vi "禹山电导率校准.vi"() -> ()   [LabVIEW 2016, in "斯坦道多参数.lvlib"]
uses:
  <vilib>/Utility/miscctls.llb/LVPointTypeDef.ctl
  <vilib>/Analysis/NI_AALBase.lvlib
  <vilib>/Analysis/NI_AALPro.lvlib
  <vilib>/Utility/config.llb/NI_LVConfig.lvlib
panel:
  out "滤波设定":dbl
  out "盐度":dbl caption="盐度测量值" format="%#.2f"
  out "通讯状态":string
  out "第二点校准值":dbl
  out "第一点校准值":dbl
  out "最小值":sgl format="%.2g"
  out "最大值":sgl format="%.2g"
  in  "校准停止":bool
  in  "校准模式":u16(ring) items=["两点校准", "单点校准"]
  in  "标液2":dbl
  in  "标液1":dbl
  out "波形图表":sgl(graph) caption="历史曲线"
  out "温度测量值":dbl caption="温度" format="%#.2f"
  out "变异系数":dbl format="%.6g"
  out "standard deviation":dbl caption="标准差" format="%0.2f"
  out "mean":dbl caption="均值" format="%0.2f"
  out "提示":string
  in  "校准启动":bool
  out "测试值":dbl format="%#.2f"
  out "电极斜率":dbl format="%#.6f"
  out "电极零点":dbl format="%#.6f"
  # "电导率电极设定"
  # "℃"
  # "μS/cm"
  # "ppt"
  # "请选择校准模式:"
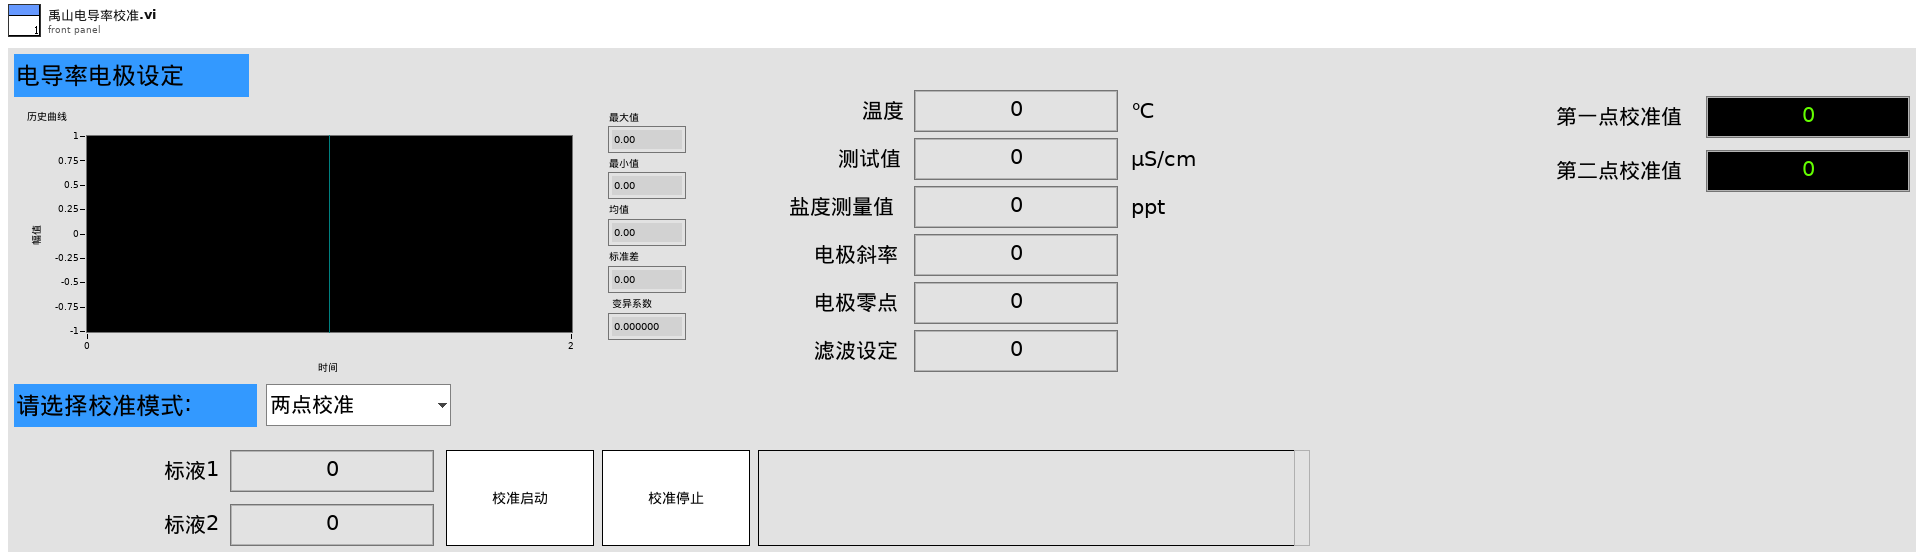
[diagram p1: front panel]
types:
  T1 = enum16{"pH", "DO", "Cond", "Turb", "ORP", "叶绿素a", "藻密度"}
  T2 = typedef "LVPointTypeDef.ctl" = cluster{"Horizontal":i16, "Vertical":i16}
  T3 = cluster{"pH":u32, "DO":u32, "Cond":u32, "Turb":u32, "叶绿素a":u32, "藻密度":u32, "ORP":u32, "COD":u32}
  T4 = typedef "NI_LVConfig.lvlib/Config Data RefNum.ctl" = refnum<k1>
  T5 = cluster{"温度测量值":sgl, "测量值":sgl, "温度偏移修正值":sgl, "信号值":sgl, "数据标识":string}
  T6 = enum8{"Enabled", "Disabled", "Disabled and Grayed Out"}
  T7 = cluster{"ph":bool, "DO":bool, "Cond":bool, "Turb":bool, "叶绿素a":bool, "藻密度":bool, "ORP":bool, "COD":bool}
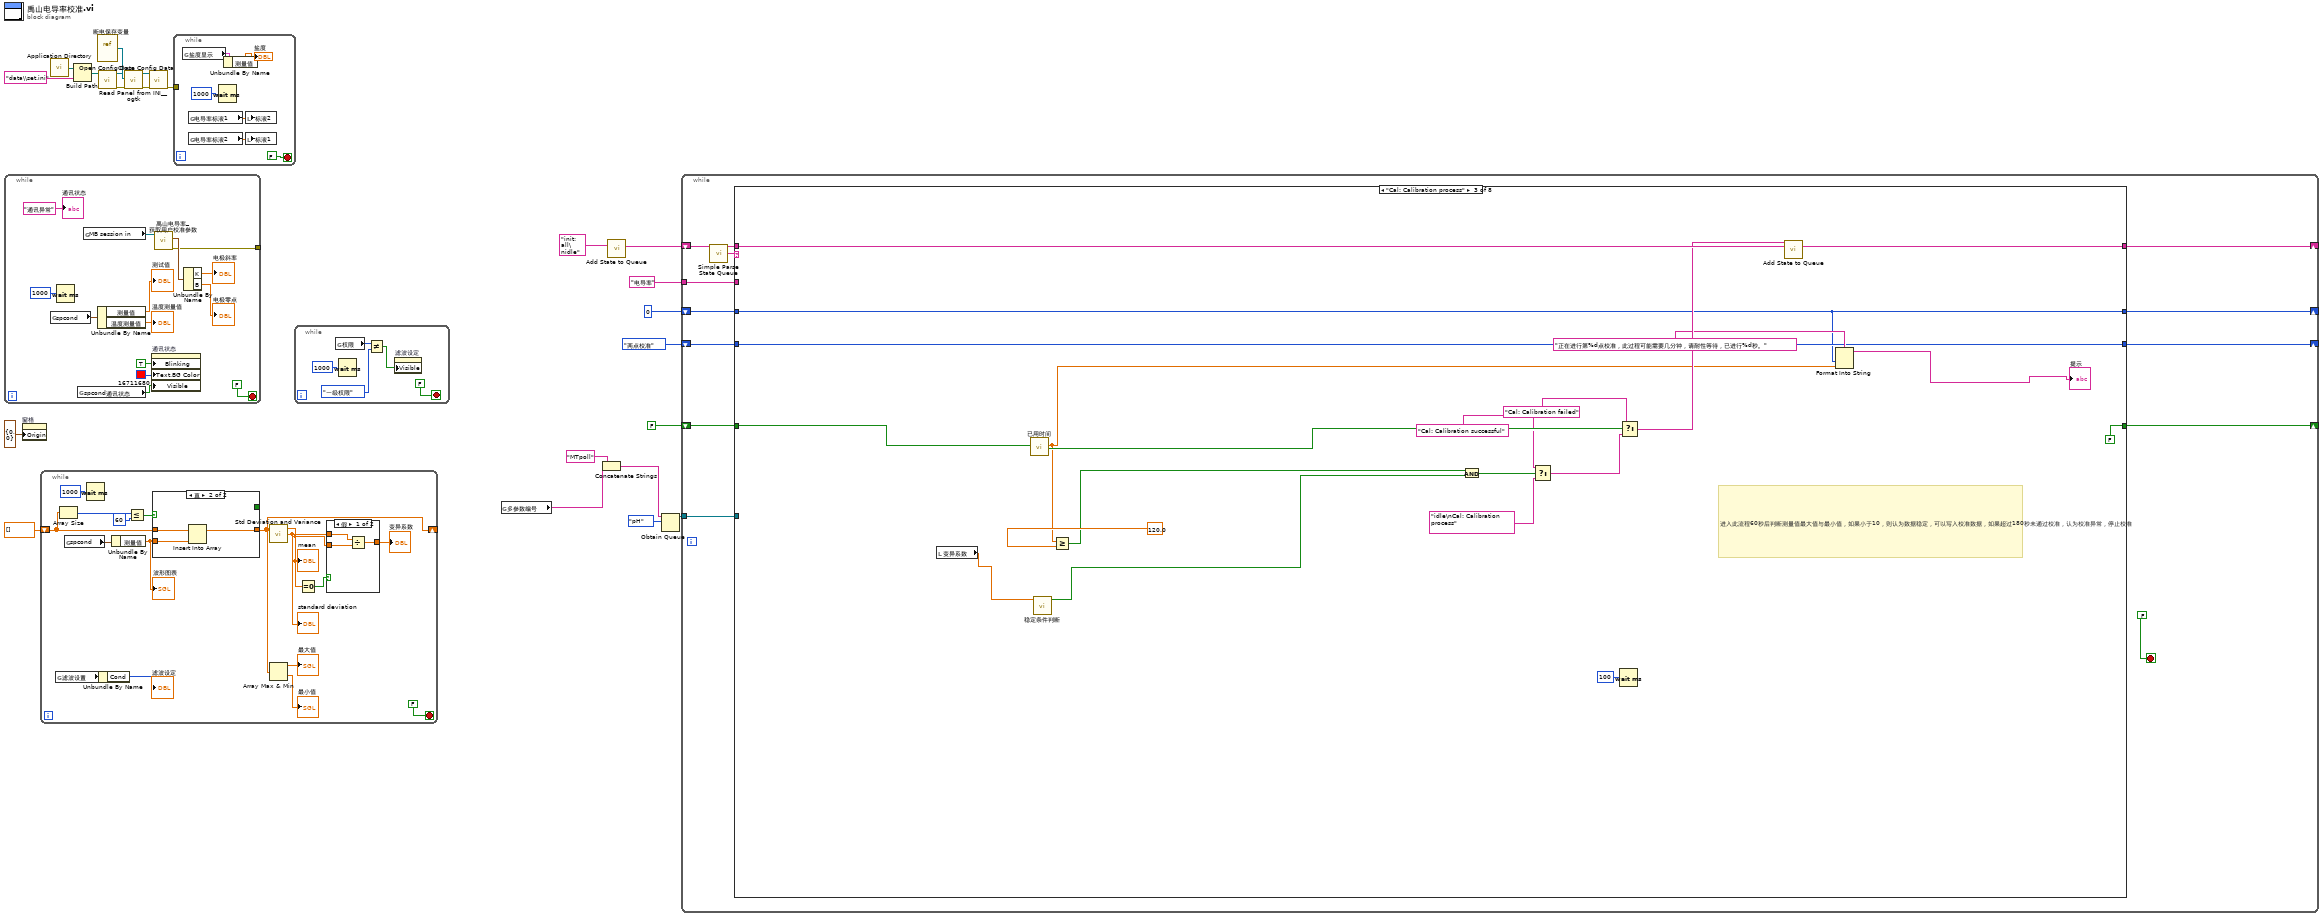
[diagram p0: block diagram]
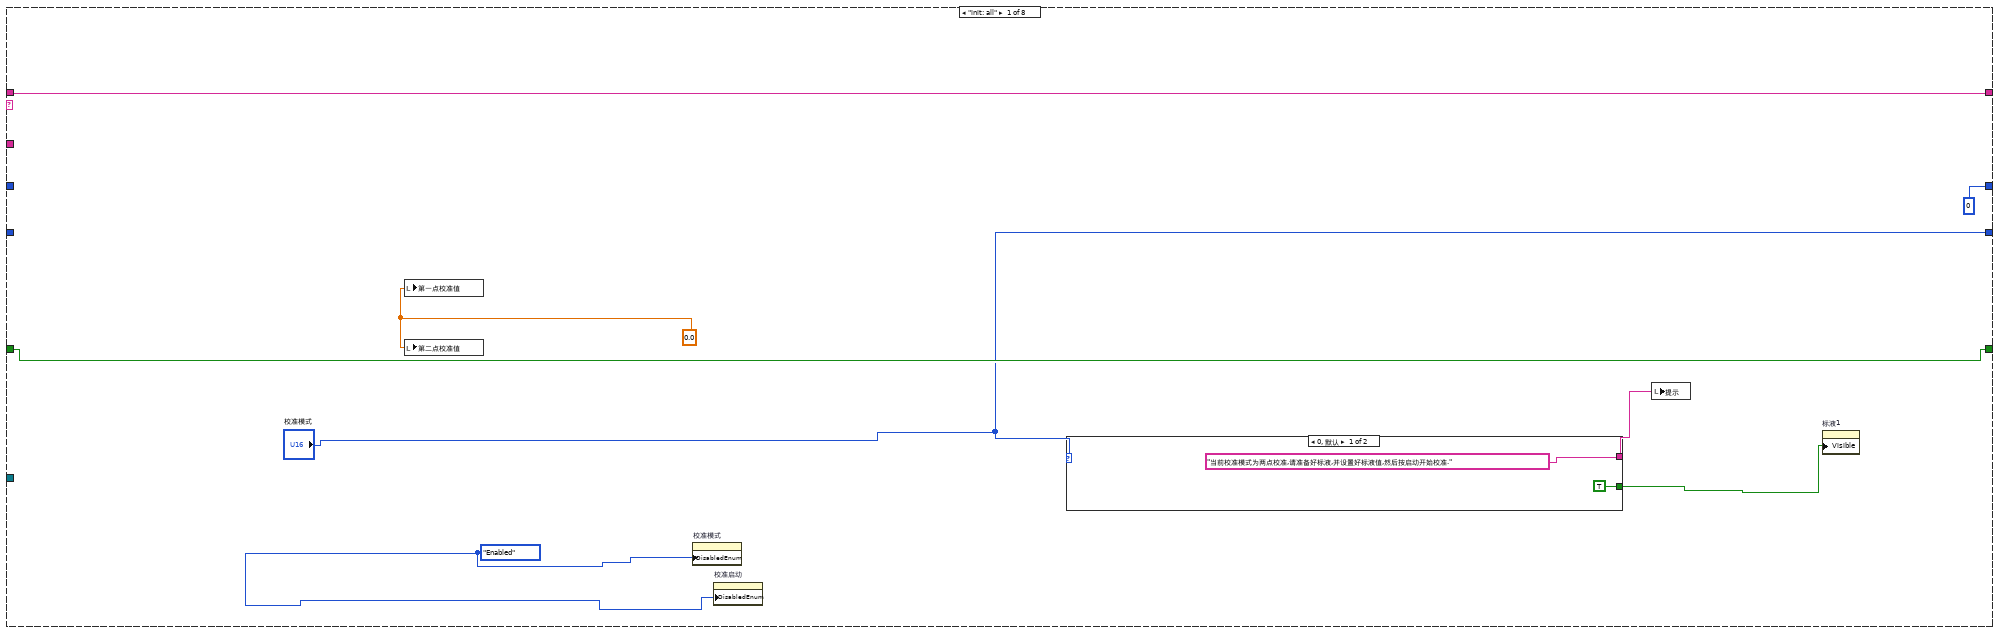
[diagram p2: hidden frame]
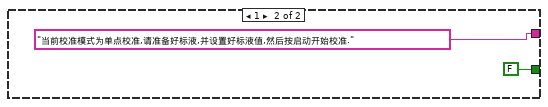
[diagram p3: hidden frame]
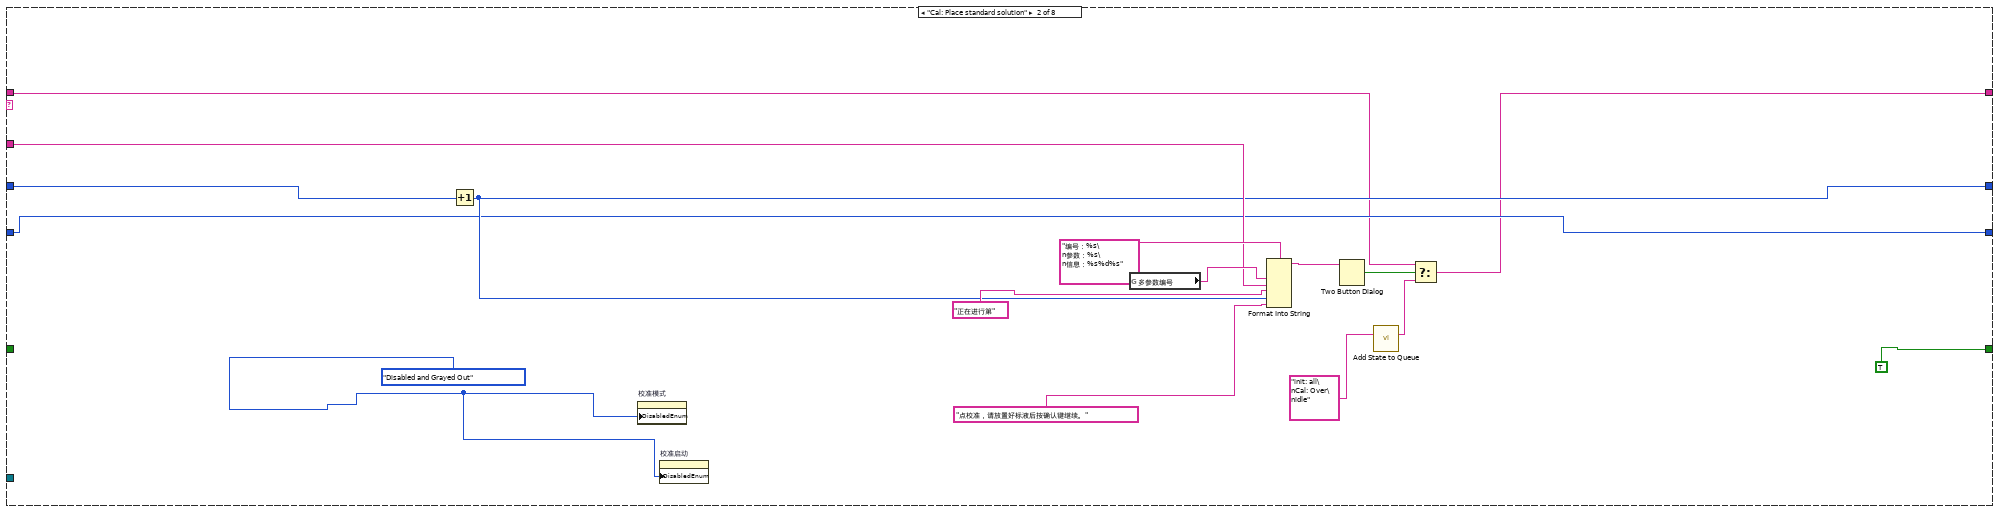
[diagram p4: hidden frame]
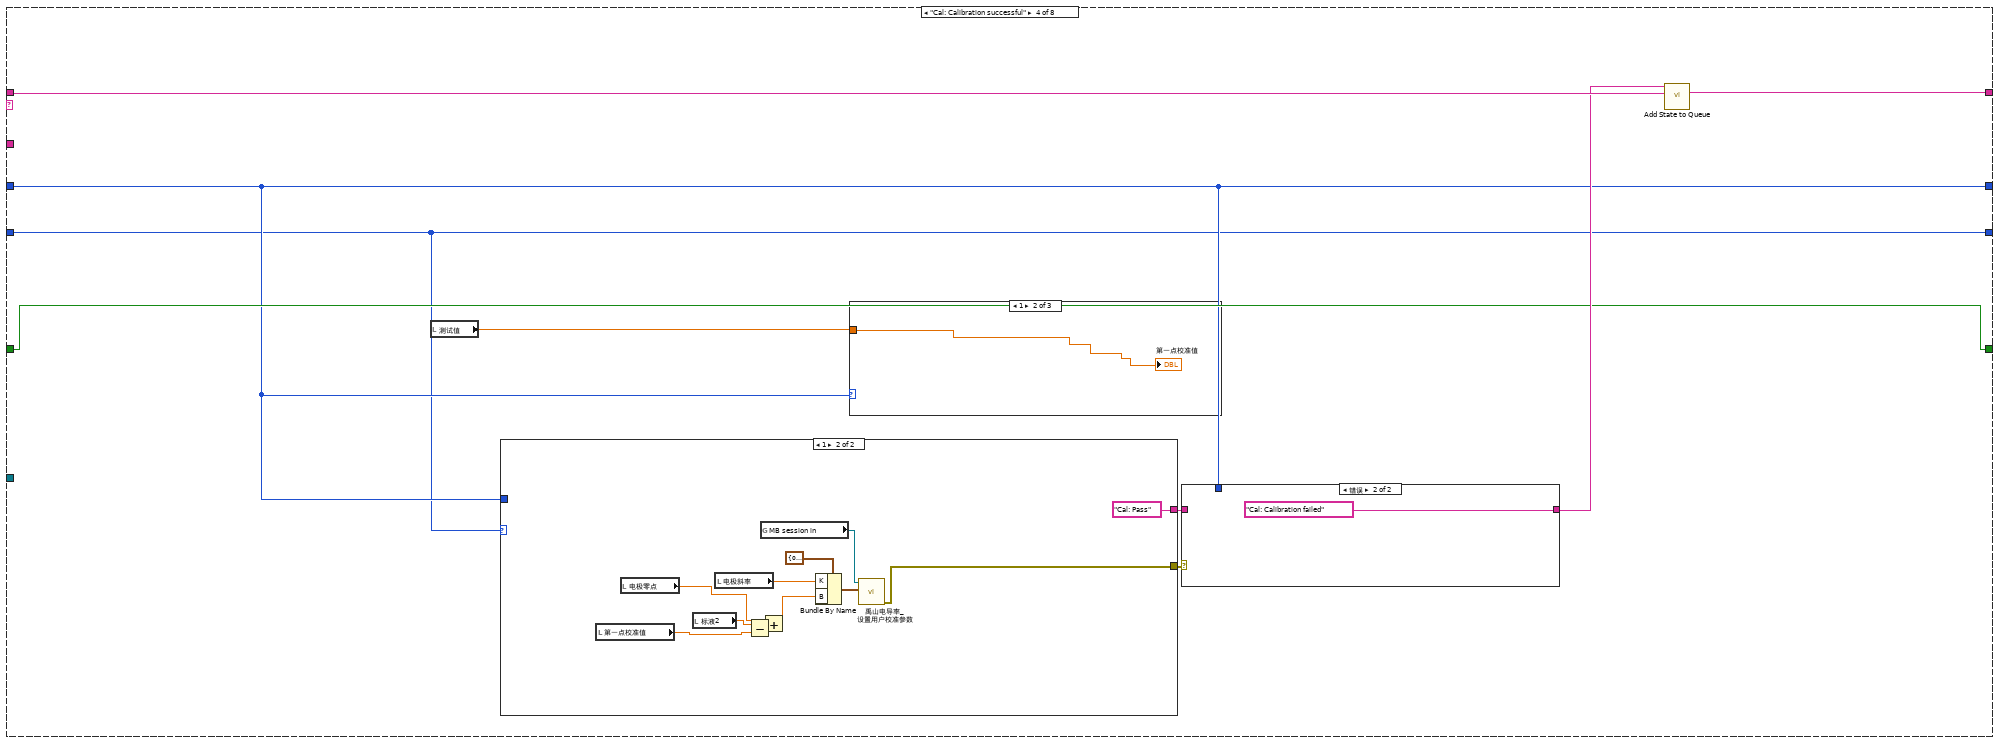
[diagram p5: hidden frame]
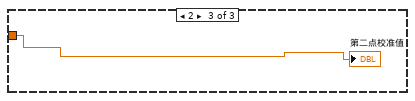
[diagram p7: hidden frame]
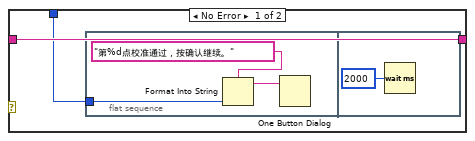
[diagram p8: hidden frame]
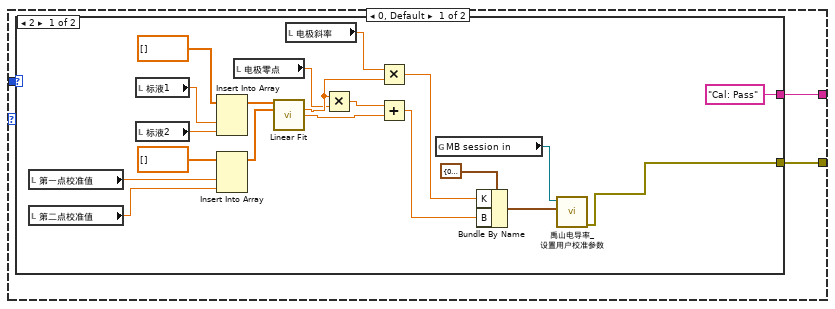
[diagram p9: hidden frame]
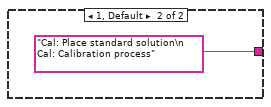
[diagram p10: hidden frame]
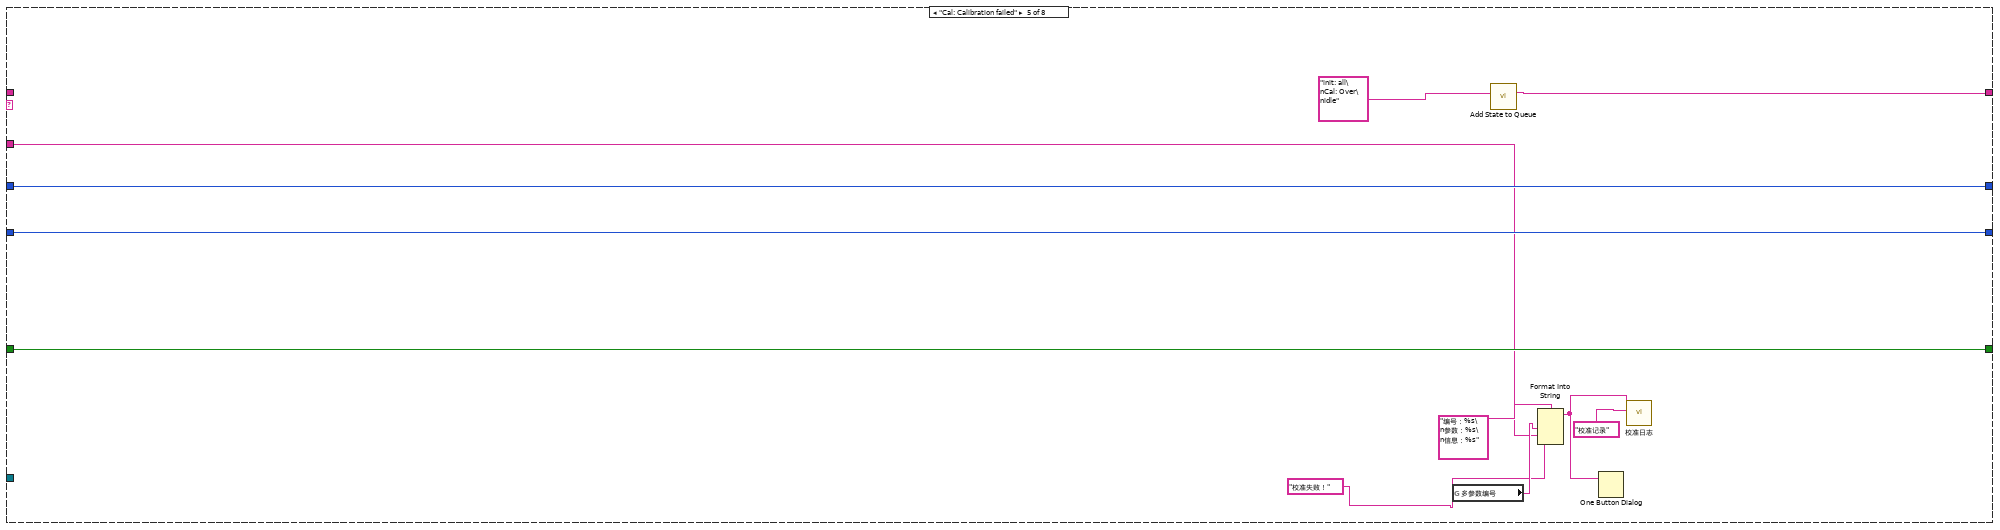
[diagram p11: hidden frame]
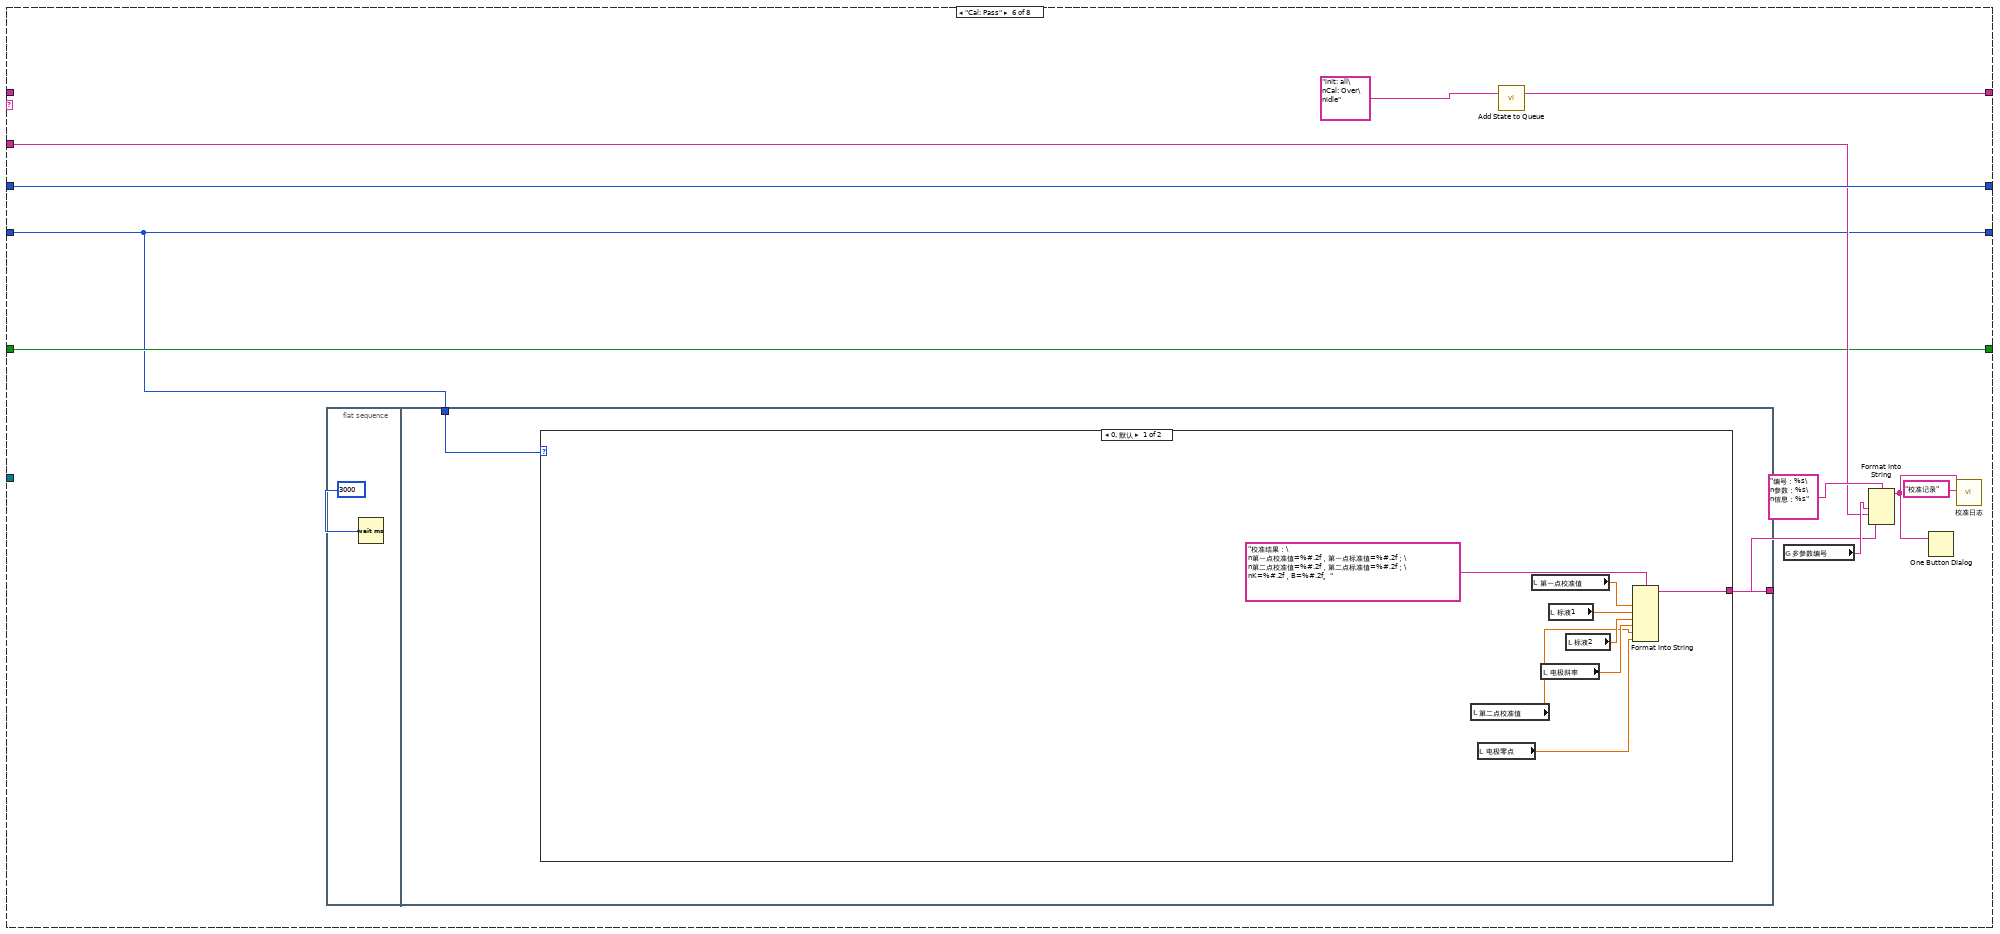
[diagram p12: hidden frame]
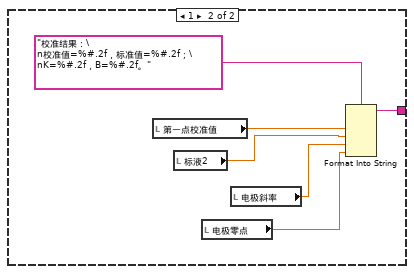
[diagram p13: hidden frame]
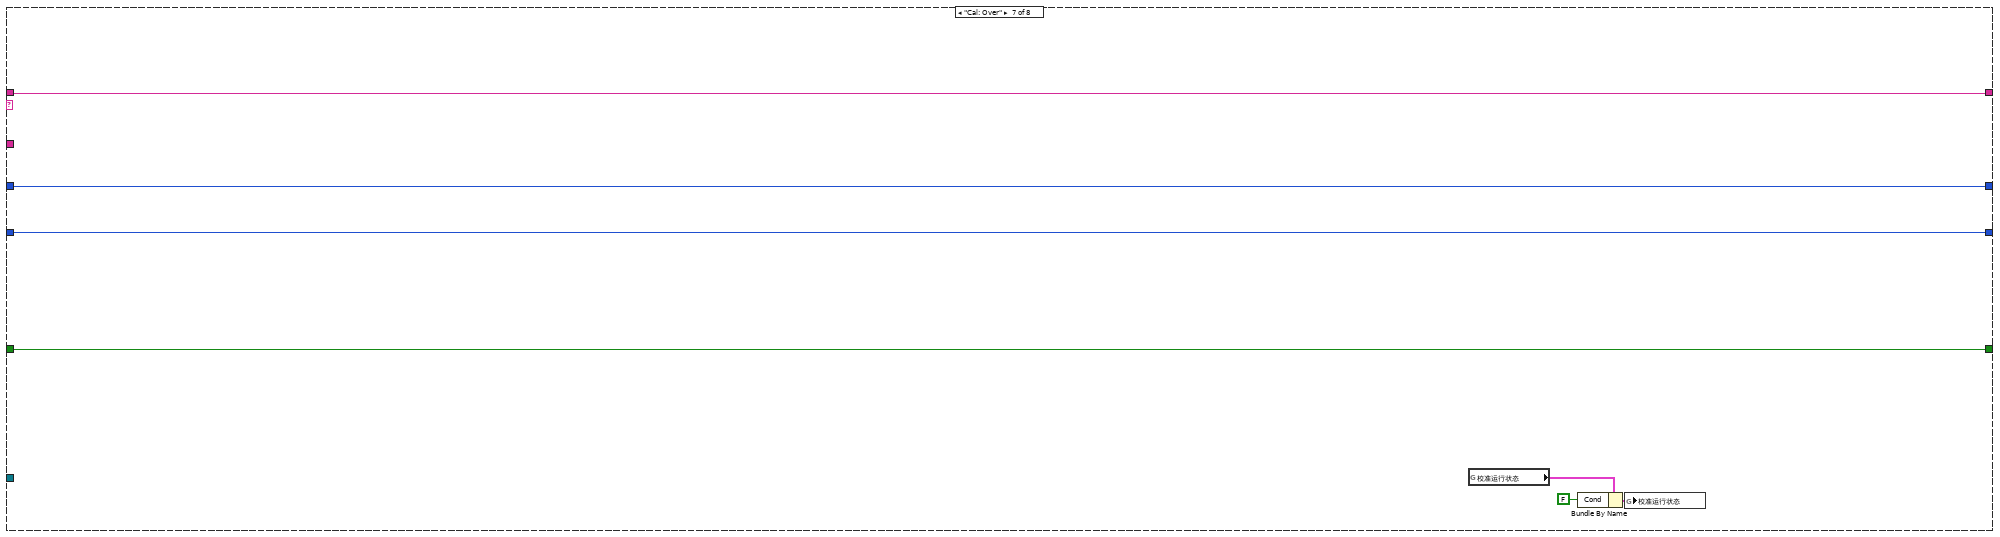
[diagram p14: hidden frame]
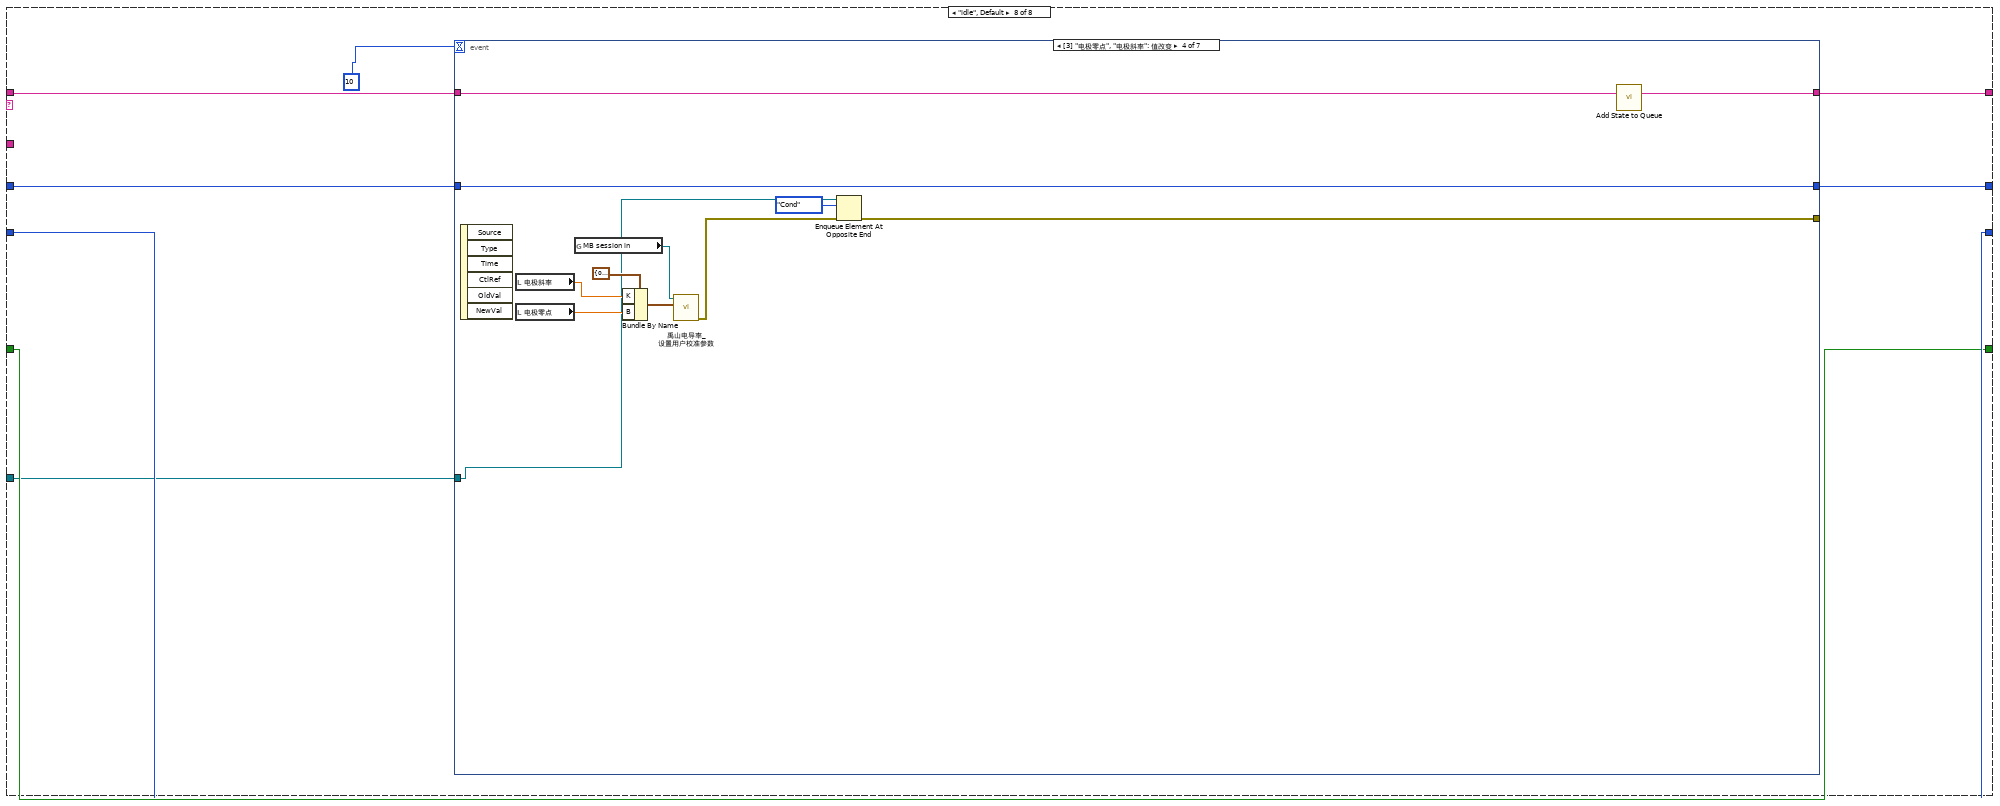
[diagram p15: hidden frame]
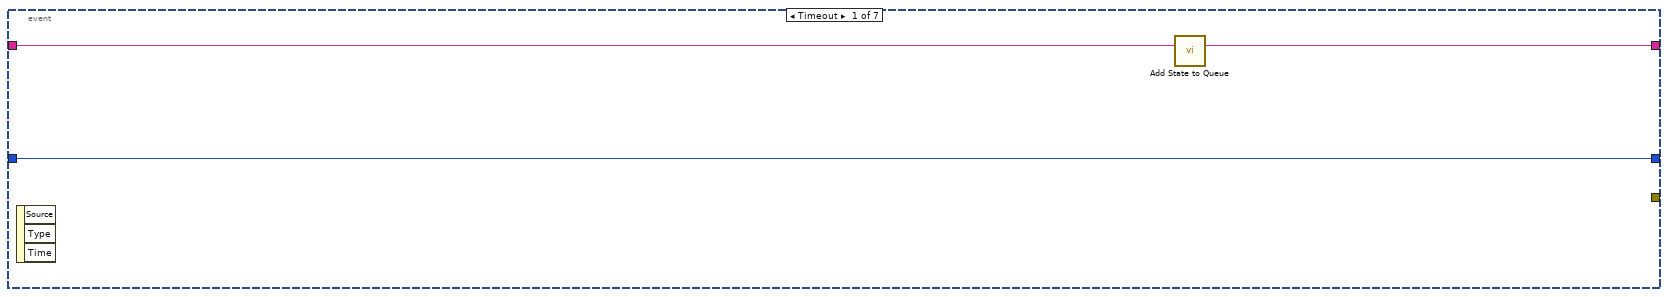
[diagram p16: hidden frame]
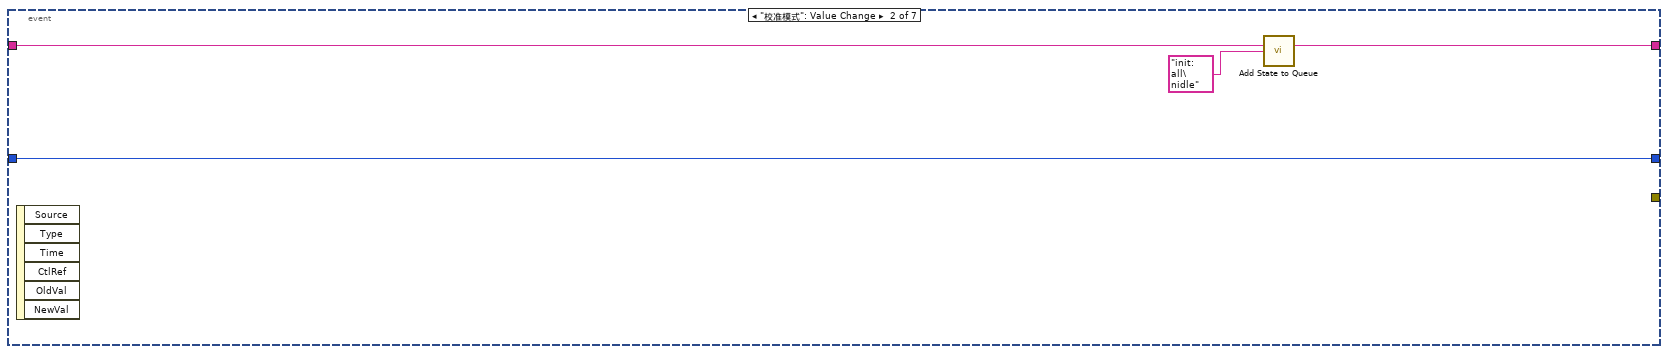
[diagram p17: hidden frame]
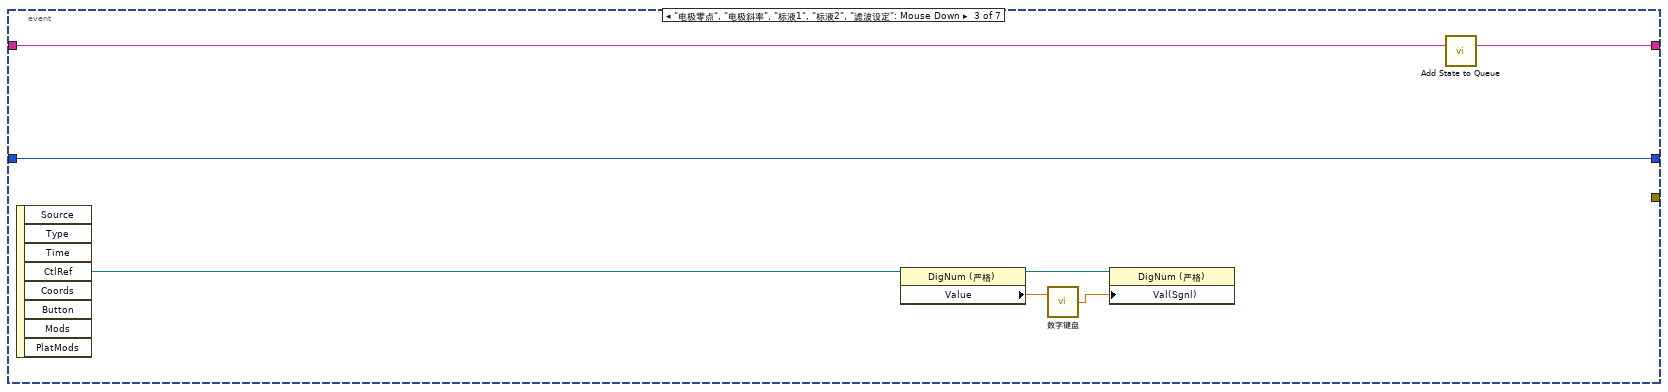
[diagram p18: hidden frame]
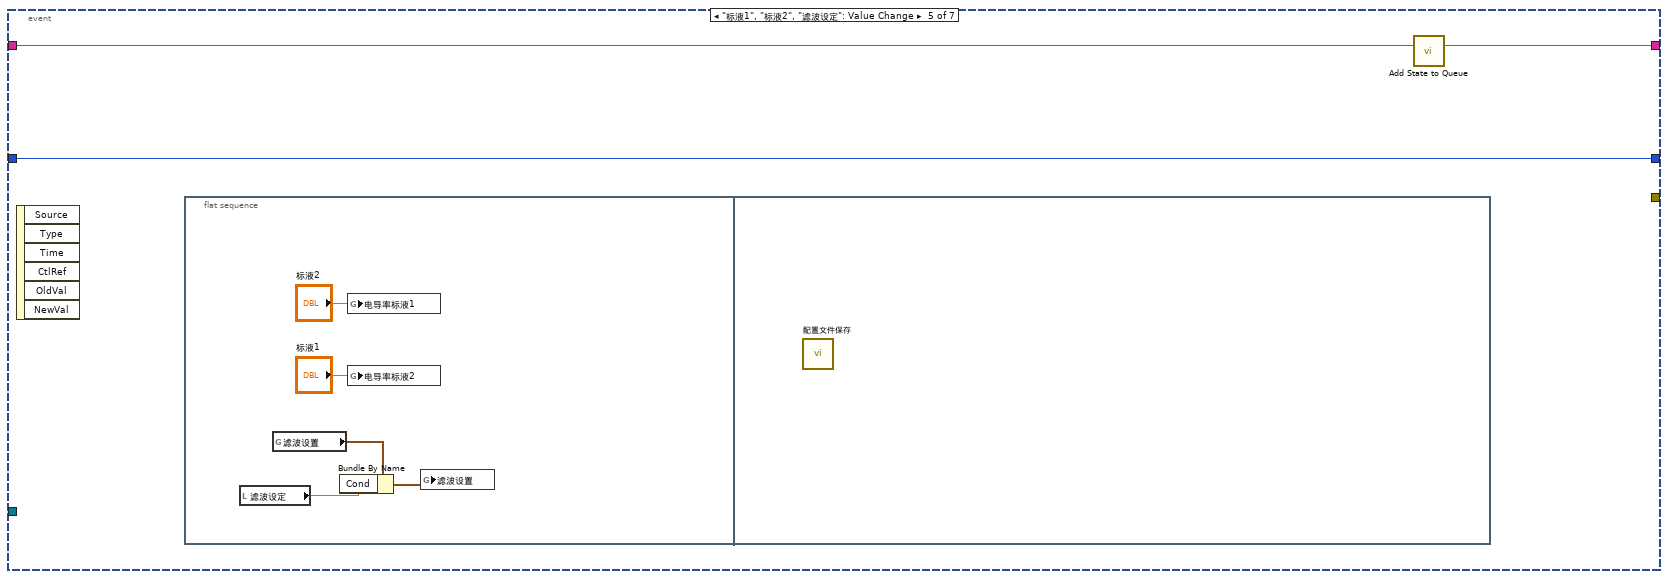
[diagram p19: hidden frame]
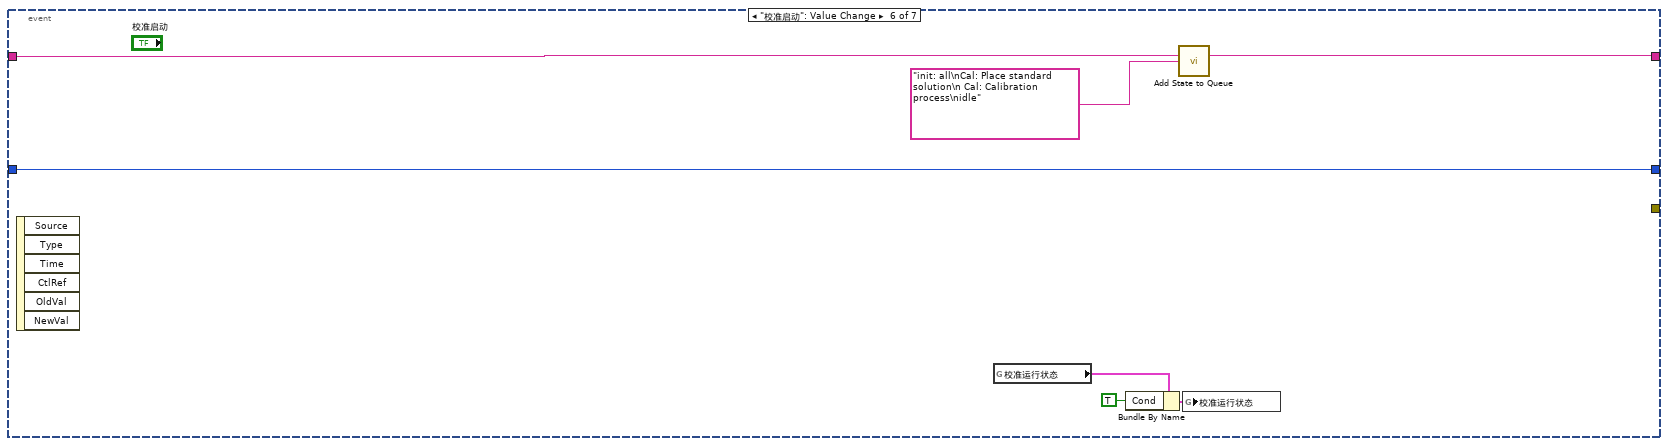
[diagram p20: hidden frame]
diagram:
  n1 = while {
    tunnel: [w31] -> _
    stop <- FALSE stop-if-true
    n2 = global read "禹山过程全局变量.vi" "spcond"() -> (w28:cluster{"温度测量值":sgl, "测量值":sgl, "错误标志":u16})
    n3 = Wait (ms)(milliseconds to wait=u32 1000 ("等待时间（毫秒）")) -> ()  [unwired: 1 out]
    n4 = global read "多参数全局变量.vi" "spcond通讯状态"() -> (w23:bool)
    n5 = global read "多参数全局变量.vi" "MB session in"() -> (w27:refnum<class "MB_Master.lvclass">)
    n6 = Unbundle By Name(w28) -> ("测量值"=→"测试值":sgl, "温度测量值"=→"温度测量值":sgl)
    n7 = property on="通讯状态" class="Str"("Blinking"=TRUE ("闪烁"), "Text.BG Color"=u32 16711680, "Visible"=w23) -> ()  [unwired: 2 in, 2 out]
    n8 = call "禹山电导率_获取用户校准参数.vi"("MB session in"=w27) -> ("error out"=w31:errorcluster, "输出值"=w34:cluster{"K":sgl, "B":sgl})  [unwired: 8 in, 1 out]
    n9 = Unbundle By Name(w34) -> ("K"=→"电极斜率":sgl, "B"=→"电极零点":sgl)
    "通讯状态" <- "通讯异常" ("当前串口")
  }
  n10 = property on="窗格" class="Pane"("Origin"=T2 {"Horizontal"=0, "Vertical"=0} ("原点")) -> ()  [unwired: 2 in, 2 out]
  n11 = while {
    shift-right: [w41] -> _
    shift-left: sgl[] [] -> [w49]
    stop <- FALSE stop-if-true
    n12 = global read "断电保存变量.vi" "滤波设置"() -> (w38:T3)
    n13 = Array Size(array=w49) -> (size(s)=w51:i32)
    n14 = global read "禹山过程全局变量.vi" "spcond"() -> (w43:cluster{"温度测量值":sgl, "测量值":sgl, "错误标志":u16})
    n15 = Wait (ms)(milliseconds to wait=u32 1000 ("等待时间（毫秒）")) -> ()  [unwired: 1 out]
    n16 = Unbundle By Name(w38) -> ("Cond"=→"滤波设定":u32)
    n17 = Unbundle By Name(w43) -> ("测量值"=w42:sgl)
    "波形图表" <- w42
    n18 = Less Or Equal?(x=w51, y=60) -> (x <= y?=w50:bool)
    n19 = case shown="真" w50 {
      tunnel: w49 -> [w62 w65]
      tunnel: w42 -> [w60 w64]
      tunnel: [w58 w63] -> w41
      tunnel: [TRUE _] -> _
      frame False {
        n20 = Replace Array Subset(array=w62, new element=w60) -> (w61:sgl[])  [unwired: 1 in]
        n21 = Rotate 1D Array(1:w61, 2:-1 ("n")) -> (0:w58:sgl[])
      }
      frame True {
        n22 = Insert Into Array(array=w65, new element=w64) -> (w63:sgl[])  [unwired: 1 in]
      }
    }
    n23 = call <vilib>:"Std Deviation and Variance.vi"("X"=w41) -> ("mean"=w44:dbl, "standard deviation"=w45:dbl)  [unwired: 1 in, 1 out]
    "standard deviation" <- w45
    "mean" <- w44
    n24 = Array Max & Min(array=w41) -> (max value=→"最大值":sgl, min value=→"最小值":sgl)  [unwired: 2 out]
    n25 = Equal To 0?(x=w44) -> (x = 0?=w48:bool)
    n26 = case shown="假" w48 {
      tunnel: w45 -> [w56 _]
      tunnel: [w55 _] -> w47
      tunnel: w44 -> [w54 _]
      frame False {
        n27 = Divide(x=w56, y=w54) -> (x/y=w55:dbl)
      }
      frame True {
      }
    }
    "变异系数" <- w47
  }
  n28 = call <vilib>:"Application Directory.vi"() -> ("Application Directory"=w17:path)
  n29 = Build Path(base path=w17, name or relative path="data\\set.ini" ("名称或相对路径")) -> (appended path=w18:path)
  n30 = vi-ref "断电保存变量.vi"() -> (w20:refnum<vi>)
  n31 = call <vilib>:"Open Config Data.vi"("configuration file path"=w18) -> ("error out"=w14:errorcluster, "refnum"=w13:T4)  [unwired: 8 in, 1 out]
  n32 = call <userlib>:"Read Panel from INI__ogtk.vi"("error in (no error)"=w14, "VI ref"=w20, "refnum"=w13) -> ("error out"=w16:errorcluster, "refnum out"=w15:T4)  [unwired: 7 in]
  n33 = call <vilib>:"Close Config Data.vi"("error in (no error)"=w16, "refnum"=w15) -> ("error out"=w12:errorcluster)  [unwired: 8 in, 1 out]
  n34 = while {
    tunnel: w12 -> [_]
    stop <- FALSE stop-if-true
    n35 = global read "多参数全局变量.vi" "盐度显示"() -> (w67:T5)
    n36 = global read "断电保存变量.vi" "电导率标液1"() -> (w68:dbl)
    n37 = global read "断电保存变量.vi" "电导率标液2"() -> (w69:dbl)
    n38 = Wait (ms)(milliseconds to wait=u32 1000 ("等待时间（毫秒）")) -> ()  [unwired: 1 out]
    n39 = Unbundle By Name(w67) -> ("测量值"=→"盐度":sgl)
    n40 = local write "标液2"(w68) -> ()
    n41 = local write "标液1"(w69) -> ()
  }
  n42 = while {
    stop <- FALSE stop-if-true
    n43 = global read "多参数全局变量.vi" "权限"() -> (w75:enum16{"一级权限", "二级权限", "三级权限"})
    n44 = Wait (ms)(milliseconds to wait=u32 1000 ("等待时间（毫秒）")) -> ()  [unwired: 1 out]
    n45 = Not Equal?(x=w75, y=enum16{"一级权限", "二级权限", "三级权限"}."一级权限") -> (x != y?=w72:bool)
    n46 = property on="滤波设定" class="DigNum (严格)"("Visible"=w72) -> ()  [unwired: 2 in, 2 out]
  }
  n47 = global read "多参数全局变量.vi" "多参数编号"() -> (w2:string)
  n48 = Concatenate Strings("MTpoll" ("名称（未命名）"), w2) -> (w4:string)
  n49 = call "Add State to Queue.vi"("State(s) In (\"\")"="init: all\nidle" ("State(s) In (\"\")")) -> ("States Out"=w10:string)  [unwired: 14 in]
  n50 = Obtain Queue(name (unnamed)=w4, element data type=T1."pH" ("枚举")) -> (queue out=w1:refnum<queue>)  [unwired: 3 in, 2 out]
  n51 = while {
    shift-right: [w85] -> _
    shift-left: w10 -> [w89]
    shift-right: [w82] -> _
    shift-left: 0 -> [w84]
    tunnel: "电导率" ("State(s) In (\"\")") -> [w83]
    shift-right: [w80] -> _
    shift-left: enum16{"两点校准", "单点校准"}."两点校准" ("校准模式") -> [w81]
    shift-right: [w78] -> _
    shift-left: FALSE -> [w79]
    tunnel: w1 -> [w77]
    stop <- FALSE stop-if-true
    n52 = call "Simple Parse State Queue.vi"("State Queue"=w89) -> ("Remain States"=w86:string, "Next State"=w87:string)  [unwired: 13 in]
    n53 = case shown="\"Cal: Calibration process\"" w87 {
      tunnel: w86 -> [w97 w105 w137 w145 _ _ w234 w245]
      tunnel: [w97 w104 w136 w144 w199 w204 w234 w244] -> w85
      tunnel: w84 -> [_ w113 w122 w140 w202 w213 w233 w242]
      tunnel: w83 -> [_ w114 _ _ w193 w209 _ _]
      tunnel: [0 w111 w122 w140 w202 w213 w233 w243] -> w82
      tunnel: w81 -> [_ w110 w123 w139 w201 w205 w232 w241]
      tunnel: ["校准模式" w110 w123 w139 w201 w205 w232 w241] -> w80
      tunnel: w79 -> [w94 _ w125 w141 w200 w208 w231 w239]
      tunnel: [w94 TRUE FALSE w141 w200 w208 w231 w239] -> w78
      tunnel: w77 -> [_ _ _ _ _ _ _ w238]
      frame "init: all" {
        w91 = T6."Enabled" ("禁用")
        w93 = 0.0 ("第一点校准值")
        n54 = local write "第一点校准值"(w93) -> ()
        n55 = local write "第二点校准值"(w93) -> ()
        n56 = property on="校准模式" class="Ring (严格)"("DisabledEnum"=w91) -> ()  [unwired: 2 in, 2 out]
        n57 = property on="校准启动" class="Bool"("DisabledEnum"=w91) -> ()  [unwired: 2 in, 2 out]
        n58 = case shown="0, 默认" "校准模式" {
          tunnel: ["当前校准模式为两点校准,请准备好标液,并设置好标液值,然后按启动开始校准." ("提示") "当前校准模式为单点校准,请准备好标液,并设置好标液值,然后按启动开始校准." ("提示")] -> w96
          tunnel: [TRUE ("可见") FALSE ("可见")] -> w90
          frame 0, Default {
          }
          frame 1 {
          }
        }
        n59 = local write "提示"(w96) -> ()
        n60 = property on="标液1" class="DigNum (严格)"("Visible"=w90) -> ()  [unwired: 2 in, 2 out]
      }
      frame "Cal: Place standard solution" {
        w103 = T6."Disabled and Grayed Out" ("禁用")
        n61 = Increment(x=w113) -> (x+1=w111:i32)
        n62 = property on="校准模式" class="Ring (严格)"("DisabledEnum"=w103) -> ()  [unwired: 2 in, 2 out]
        n63 = property on="校准启动" class="Bool"("DisabledEnum"=w103) -> ()  [unwired: 2 in, 2 out]
        n64 = global read "多参数全局变量.vi" "多参数编号"() -> (w116:string)
        n65 = Format Into String(format string="编号：%s\n参数：%s\n信息：%s%d%s" ("格式字符串"), w116, w114, "正在进行第" ("消息"), w111, "点校准，请放置好标液后按确认键继续。" ("消息")) -> (resulting string=w108:string)  [unwired: 2 in, 1 out]
        n66 = Two Button Dialog(message=w108) -> (T button?=w107:bool)  [unwired: 2 in]
        n67 = call "Add State to Queue.vi"("State(s) In (\"\")"="init: all\nCal: Over\nidle" ("State(s) In (\"\")")) -> ("States Out"=w106:string)  [unwired: 14 in]
        n68 = Select(t=w105, s=w107, f=w106) -> (s? t:f=w104:string)
      }
      frame "Cal: Calibration process" {
        # "进入此流程60秒后判断测量值最大值与最小值，如果小于10，则认为数据稳定，可以写入校准数据，如果超过180秒未通过校准，认为校准异常，停止校准"
        n69 = local read "变异系数"() -> (w119:dbl)
        n70 = call "已用时间"("Reset"=w125) -> ("Elapsed Time (s)"=w121:dbl, "Time has Elapsed"=w138:bool)  [unwired: 11 in, 6 out]
        n71 = call "稳定条件判断.vi"("变异系数"=w119) -> ("布尔"=w118:bool)  [unwired: 10 in]
        n72 = Greater Or Equal?(x=w121, y=120.0) -> (x >= y?=w133:bool)
        n73 = And(x=w133, y=w118) -> (x .and. y?=w130:bool)
        n74 = Select(t="Cal: Calibration successful" ("State(s) In (\"\")"), s=w130, f="idle\nCal: Calibration process" ("State(s) In (\"\")")) -> (s? t:f=w129:string)
        n75 = Wait (ms)(milliseconds to wait=u32 100 ("等待时间（毫秒）")) -> ()  [unwired: 1 out]
        n76 = Select(t="Cal: Calibration failed" ("State(s) In (\"\")"), s=w138, f=w129) -> (s? t:f=w128:string)
        n77 = call "Add State to Queue.vi"("State(s) In Front (\"\")"=w128, "State(s) In (\"\")"=w137) -> ("States Out"=w136:string)  [unwired: 13 in]
        n78 = Format Into String(format string="正在进行第%d点校准，此过程可能需要几分钟，请耐性等待，已进行%d秒。" ("格式字符串"), w122, w121) -> (resulting string=→"提示":string)  [unwired: 2 in, 1 out]
      }
      frame "Cal: Calibration successful" {
        n79 = local read "测试值"() -> (w142:dbl)
        n80 = case shown="1" w139 {
          tunnel: [w159 w181] -> w147
          tunnel: [w158 "Cal: Pass" ("State(s) In (\"\")")] -> w146
          tunnel: w140 -> [w157 _]
          frame 0, Default {
            n81 = case shown="2" w157 {
              tunnel: [w160 _] -> w159
              tunnel: ["Cal: Pass" ("State(s) In (\"\")") "Cal: Place standard solution\n Cal: Calibration process" ("State(s) In (\"\")")] -> w158
              frame 2 {
                n82 = local read "第一点校准值"() -> (w177:dbl)
                n83 = local read "第二点校准值"() -> (w176:dbl)
                n84 = local read "标液1"() -> (w174:dbl)
                n85 = local read "标液2"() -> (w173:dbl)
                n86 = Insert Into Array(array=dbl[] [] ("Weight"), new element #1=w174, new element #2=w173) -> (w172:dbl[])  [unwired: 1 in]
                n87 = Insert Into Array(array=dbl[] [] ("Weight"), new element #1=w177, new element #2=w176) -> (w171:dbl[])  [unwired: 1 in]
                n88 = local read "电极零点"() -> (w164:dbl)
                n89 = call <vilib>:"Linear Fit.vi"("Y"=w172, "X"=w171) -> ("slope"=w165:dbl, "intercept"=w162:dbl)  [unwired: 9 in, 3 out]
                n90 = local read "电极斜率"() -> (w167:dbl)
                n91 = Multiply(x=w165, y=w164) -> (x*y=w163:dbl)
                n92 = Multiply(x=w167, y=w165) -> (x*y=w166:dbl)
                n93 = Add(x=w163, y=w162) -> (x+y=w161:dbl)
                n94 = global read "多参数全局变量.vi" "MB session in"() -> (w170:refnum<class "MB_Master.lvclass">)
                n95 = Bundle By Name(cluster=cluster{"K":sgl, "B":sgl} {"K"=0.0, "B"=0.0} ("用户校准参数"), "K"=w166, "B"=w161) -> (w169:cluster{"K":sgl, "B":sgl})
                n96 = call "禹山电导率_设置用户校准参数.vi"("用户校准参数"=w169, "MB session in"=w170) -> ("error out"=w160:errorcluster)  [unwired: 8 in, 1 out]
              }
              frame 1, Default {
              }
            }
          }
          frame 1 {
            n97 = local read "第一点校准值"() -> (w186:dbl)
            n98 = local read "电极零点"() -> (w182:dbl)
            n99 = local read "标液2"() -> (w185:dbl)
            n100 = local read "电极斜率"() -> (w187:dbl)
            n101 = Subtract(x=w185, y=w186) -> (x-y=w184:dbl)
            n102 = global read "多参数全局变量.vi" "MB session in"() -> (w190:refnum<class "MB_Master.lvclass">)
            n103 = Add(x=w182, y=w184) -> (x+y=w183:dbl)
            n104 = Bundle By Name(cluster=cluster{"K":sgl, "B":sgl} {"K"=0.0, "B"=0.0} ("用户校准参数"), "K"=w187, "B"=w183) -> (w189:cluster{"K":sgl, "B":sgl})
            n105 = call "禹山电导率_设置用户校准参数.vi"("用户校准参数"=w189, "MB session in"=w190) -> ("error out"=w181:errorcluster)  [unwired: 8 in, 1 out]
          }
        }
        n106 = case shown="1" w140 {
          tunnel: w142 -> [_ w148 w149]
          frame 0, Default {
          }
          frame 1 {
            "第一点校准值" <- w148
          }
          frame 2 {
            "第二点校准值" <- w149
          }
        }
        n107 = case shown="错误" w147 {
          tunnel: w146 -> [w151 _]
          tunnel: [w151 "Cal: Calibration failed" ("State(s) In (\"\")")] -> w143
          tunnel: w140 -> [w150 _]
          frame No Error {
            n108 = flat-sequence {
              tunnel: w150 -> [w152]
              frame #0 {
                n109 = Format Into String(format string="第%d点校准通过，按确认继续。" ("格式字符串"), w152) -> (resulting string=w154:string)  [unwired: 2 in, 1 out]
                n110 = One Button Dialog(message=w154) -> ()  [unwired: 1 in, 1 out]
              }
              frame #1 {
                n111 = Wait (ms)(milliseconds to wait=u32 2000 ("等待时间（毫秒）")) -> ()  [unwired: 1 out]
              }
            }
          }
          frame Error {
          }
        }
        n112 = call "Add State to Queue.vi"("State(s) In Front (\"\")"=w143, "State(s) In (\"\")"=w145) -> ("States Out"=w144:string)  [unwired: 13 in]
      }
      frame "Cal: Calibration failed" {
        n113 = global read "多参数全局变量.vi" "多参数编号"() -> (w196:string)
        n114 = call "Add State to Queue.vi"("State(s) In (\"\")"="init: all\nCal: Over\nidle" ("State(s) In (\"\")")) -> ("States Out"=w199:string)  [unwired: 14 in]
        n115 = Format Into String(format string="编号：%s\n参数：%s\n信息：%s" ("格式字符串"), w196, w193, "校准失败！" ("消息")) -> (resulting string=w195:string)  [unwired: 2 in, 1 out]
        n116 = One Button Dialog(message=w195) -> ()  [unwired: 1 in, 1 out]
        n117 = call "校准日志.vi"("table"="校准记录", "日志信息"=w195) -> ()  [unwired: 9 in, 1 out]
      }
      frame "Cal: Pass" {
        n118 = flat-sequence {
          tunnel: [w216] -> w206
          tunnel: w205 -> [w215]
          frame #0 {
            n119 = Wait (ms)(milliseconds to wait=u32 3000 ("等待时间（毫秒）")) -> ()  [unwired: 1 out]
          }
          frame #1 {
            n120 = case shown="0, 默认" w215 {
              tunnel: [w224 w230] -> w216
              frame 0, Default {
                n121 = local read "第二点校准值"() -> (w218:dbl)
                n122 = local read "电极零点"() -> (w217:dbl)
                n123 = local read "第一点校准值"() -> (w222:dbl)
                n124 = local read "电极斜率"() -> (w219:dbl)
                n125 = local read "标液1"() -> (w223:dbl)
                n126 = local read "标液2"() -> (w220:dbl)
                n127 = Format Into String(format string="校准结果：\n第一点校准值=%#.2f，第一点标准值=%#.2f；\n第二点校准值=%#.2f，第二点标准值=%#.2f；\nK=%#.2f，B=%#.2f。" ("提示"), w222, w223, w220, w219, w218, w217) -> (resulting string=w224:string)  [unwired: 2 in, 1 out]
              }
              frame 1 {
                n128 = local read "第一点校准值"() -> (w229:dbl)
                n129 = local read "标液2"() -> (w227:dbl)
                n130 = local read "电极零点"() -> (w225:dbl)
                n131 = local read "电极斜率"() -> (w226:dbl)
                n132 = Format Into String(format string="校准结果：\n校准值=%#.2f，标准值=%#.2f；\nK=%#.2f，B=%#.2f。" ("提示"), w229, w227, w226, w225) -> (resulting string=w230:string)  [unwired: 2 in, 1 out]
              }
            }
          }
        }
        n133 = call "Add State to Queue.vi"("State(s) In (\"\")"="init: all\nCal: Over\nidle" ("State(s) In (\"\")")) -> ("States Out"=w204:string)  [unwired: 14 in]
        n134 = global read "多参数全局变量.vi" "多参数编号"() -> (w210:string)
        n135 = Format Into String(format string="编号：%s\n参数：%s\n信息：%s" ("格式字符串"), w210, w209, w206) -> (resulting string=w207:string)  [unwired: 2 in, 1 out]
        n136 = One Button Dialog(message=w207) -> ()  [unwired: 1 in, 1 out]
        n137 = call "校准日志.vi"("table"="校准记录", "日志信息"=w207) -> ()  [unwired: 9 in, 1 out]
      }
      frame "Cal: Over" {
        n138 = global read "多参数全局变量.vi" "校准运行状态"() -> (w236:T7)
        n139 = Bundle By Name(cluster=w236, "Cond"=FALSE) -> (w237:T7)
        n140 = global write "多参数全局变量.vi" "校准运行状态"(w237) -> ()
      }
      frame "idle", Default {
        n141 = event shown="[3] \"电极零点\", \"电极斜率\": 值改变" {
          selector: _ -> [_ _ _ _ _ _ _]
          dyn-events: _ -> [_ _ _ _ _ _ _]
          timeout: 10 -> [_ _ _ _ _ _ _]
          tunnel: [_ _ _ w262 _ _ _] -> _
          tunnel: w245 -> [w248 w252 w257 w263 w272 w286 _]
          tunnel: [w247 w251 w258 w270 w273 w285 w288] -> w244
          tunnel: [w246 w249 w259 w271 w274 w283 w289] -> w243
          tunnel: w242 -> [w246 w249 w259 w271 w274 w283 w289]
          tunnel: w238 -> [_ _ _ w261 _ _ _]
          event Timeout {
            n142 = event-data() -> ()  [unwired: 1 in, 3 out]
            n143 = call "Add State to Queue.vi"("State(s) In (\"\")"=w248) -> ("States Out"=w247:string)  [unwired: 14 in]
          }
          event "校准模式": Value Change {
            n144 = event-data() -> ()  [unwired: 1 in, 6 out]
            n145 = call "Add State to Queue.vi"("State(s) In (\"\")"=w252, "State(s) At Back (\"\")"="init: all\nidle" ("State(s) In (\"\")")) -> ("States Out"=w251:string)  [unwired: 13 in]
          }
          event "电极零点", "电极斜率", "标液1", "标液2", "滤波设定": Mouse Down {
            n146 = event-data() -> ("CtlRef"=w256:refnum<vi>)  [unwired: 1 in, 7 out]
            n147 = property class="DigNum (严格)"(reference=w256) -> (reference out=w253:refnum<vi>, "Value"=w254:dbl)  [unwired: 1 in, 1 out]
            n148 = call "数字键盘.vi"("OldNumber"=w254) -> ("NewNumber"=w255:dbl)  [unwired: 1 in]
            n149 = property class="DigNum (严格)"(reference=w253, "Val(Sgnl)"=w255) -> ()  [unwired: 1 in, 2 out]
            n150 = call "Add State to Queue.vi"("State(s) In (\"\")"=w257) -> ("States Out"=w258:string)  [unwired: 14 in]
          }
          event "电极零点", "电极斜率": Value Change {
            n151 = event-data() -> ()  [unwired: 1 in, 6 out]
            n152 = local read "电极斜率"() -> (w267:dbl)
            n153 = local read "电极零点"() -> (w266:dbl)
            n154 = global read "多参数全局变量.vi" "MB session in"() -> (w265:refnum<class "MB_Master.lvclass">)
            n155 = Bundle By Name(cluster=cluster{"K":sgl, "B":sgl} {"K"=0.0, "B"=0.0} ("用户校准参数"), "K"=w267, "B"=w266) -> (w268:cluster{"K":sgl, "B":sgl})
            n156 = call "禹山电导率_设置用户校准参数.vi"("用户校准参数"=w268, "MB session in"=w265) -> ("error out"=w264:errorcluster)  [unwired: 8 in, 1 out]
            n157 = Enqueue Element At Opposite End(queue=w261, element=T1."Cond" ("元素"), error in (no error)=w264) -> (error out=w262:errorcluster)  [unwired: 1 in, 2 out]
            n158 = call "Add State to Queue.vi"("State(s) In (\"\")"=w263) -> ("States Out"=w270:string)  [unwired: 14 in]
          }
          event "标液1", "标液2", "滤波设定": Value Change {
            n159 = event-data() -> ()  [unwired: 1 in, 6 out]
            n160 = flat-sequence {
              frame #0 {
                n161 = local read "滤波设定"() -> (w275:dbl)
                n162 = global read "断电保存变量.vi" "滤波设置"() -> (w277:T3)
                n163 = Bundle By Name(cluster=w277, "Cond"=w275) -> (w276:T3)
                n164 = global write "断电保存变量.vi" "电导率标液1"("标液2") -> ()
                n165 = global write "断电保存变量.vi" "电导率标液2"("标液1") -> ()
                n166 = global write "断电保存变量.vi" "滤波设置"(w276) -> ()
              }
              frame #1 {
                n167 = call "配置文件保存.vi"() -> ()  [unwired: 12 in]
              }
            }
            n168 = call "Add State to Queue.vi"("State(s) In (\"\")"=w272) -> ("States Out"=w273:string)  [unwired: 14 in]
          }
          event "校准启动": Value Change {
            n169 = event-data() -> ()  [unwired: 1 in, 6 out]
            n170 = global read "多参数全局变量.vi" "校准运行状态"() -> (w281:T7)
            n171 = Bundle By Name(cluster=w281, "Cond"=TRUE) -> (w282:T7)
            n172 = call "Add State to Queue.vi"("State(s) In (\"\")"=w286, "State(s) At Back (\"\")"="init: all\nCal: Place standard solution\n Cal: Calibration process\nidle" ("State(s) In (\"\")")) -> ("States Out"=w285:string)  [unwired: 13 in]
            n173 = global write "多参数全局变量.vi" "校准运行状态"(w282) -> ()
          }
          event "校准停止": Value Change {
            n174 = event-data() -> ()  [unwired: 1 in, 6 out]
            n175 = call "Add State to Queue.vi"("State(s) In (\"\")"="init: all\nCal: Over\nidle" ("State(s) In (\"\")")) -> ("States Out"=w288:string)  [unwired: 14 in]
          }
        }
      }
    }
  }
